vi "NewDefenderNormal.vi"(6 "Defensores":u32[](array[numeric]), 7 "total":i32, 8 "Numeric":i32, 9 "Field Size in":T3, 10 "balls":T4[](array[typedef]), 11 "Our Robot in":T1) -> (2 "Robot out":T1)   [LabVIEW 2016]
uses:
  Core/AI Robot.ctl
  Functions Enum.ctl
  Core/AI Ball.ctl
  Core/Field Size.ctl
panel:
  in  "d":dbl=110.0
  in  "min dist to kick":dbl=150.0 format="%#_13g"
  in  "D max":dbl=500.0
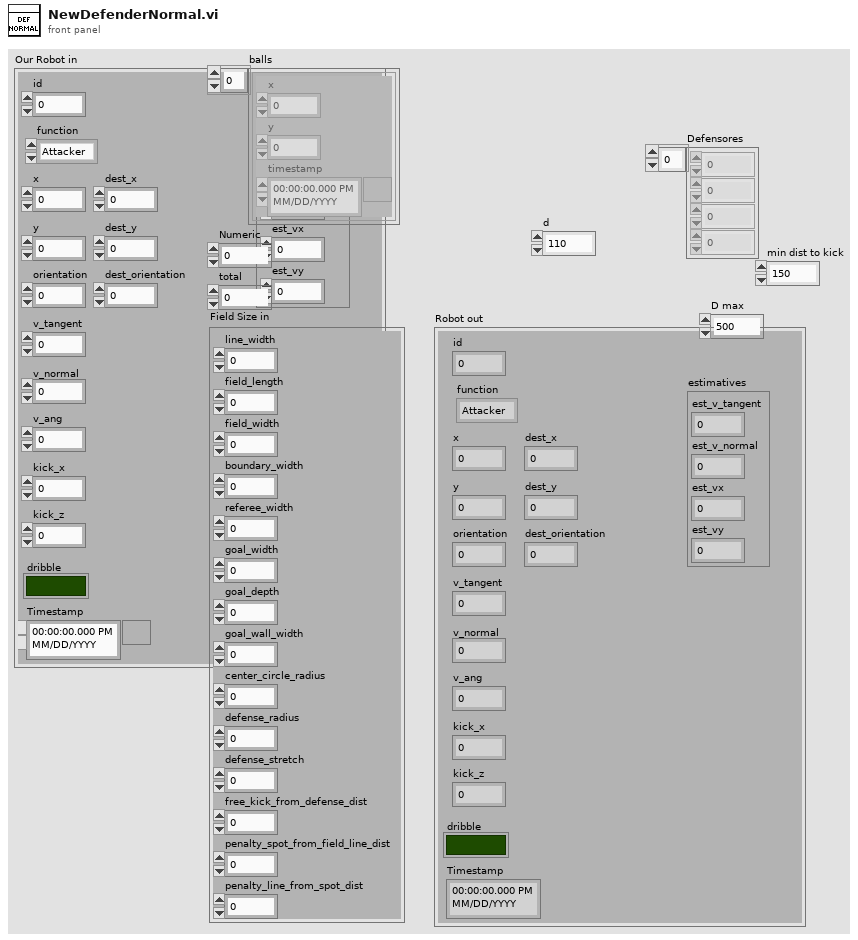
[diagram p1: front panel]
types:
  T1 = typedef "AI Robot.ctl" = cluster{"id":u32, "function":T2, "x":dbl, "y":dbl, "orientation":dbl, "v_tangent":dbl, "v_normal":dbl, "v_ang":dbl, "kick_x":dbl, "kick_z":dbl, "dribble":bool, "Timestamp":timestamp, "dest_x":dbl, "dest_y":dbl, "dest_orientation":dbl, "estimatives":cluster{"est_v_tangent":dbl, "est_v_normal":dbl, "est_vx":dbl, "est_vy":dbl}}
  T2 = typedef "Functions Enum.ctl" = enum16{"Attacker", "Goalie", "Defender", "Striker", "Goto 0", "Dummy", "ZigZag"}
  T3 = typedef "Field Size.ctl" = cluster{"line_width":u32, "field_length":u32, "field_width":u32, "boundary_width":u32, "referee_width":u32, "goal_width":u32, "goal_depth":u32, "goal_wall_width":u32, "center_circle_radius":u32, "defense_radius":u32, "defense_stretch":u32, "free_kick_from_defense_dist":u32, "penalty_spot_from_field_line_dist":u32, "penalty_line_from_spot_dist":u32}
  T4 = typedef "AI Ball.ctl" = cluster{"x":dbl, "y":dbl, "timestamp":timestamp}
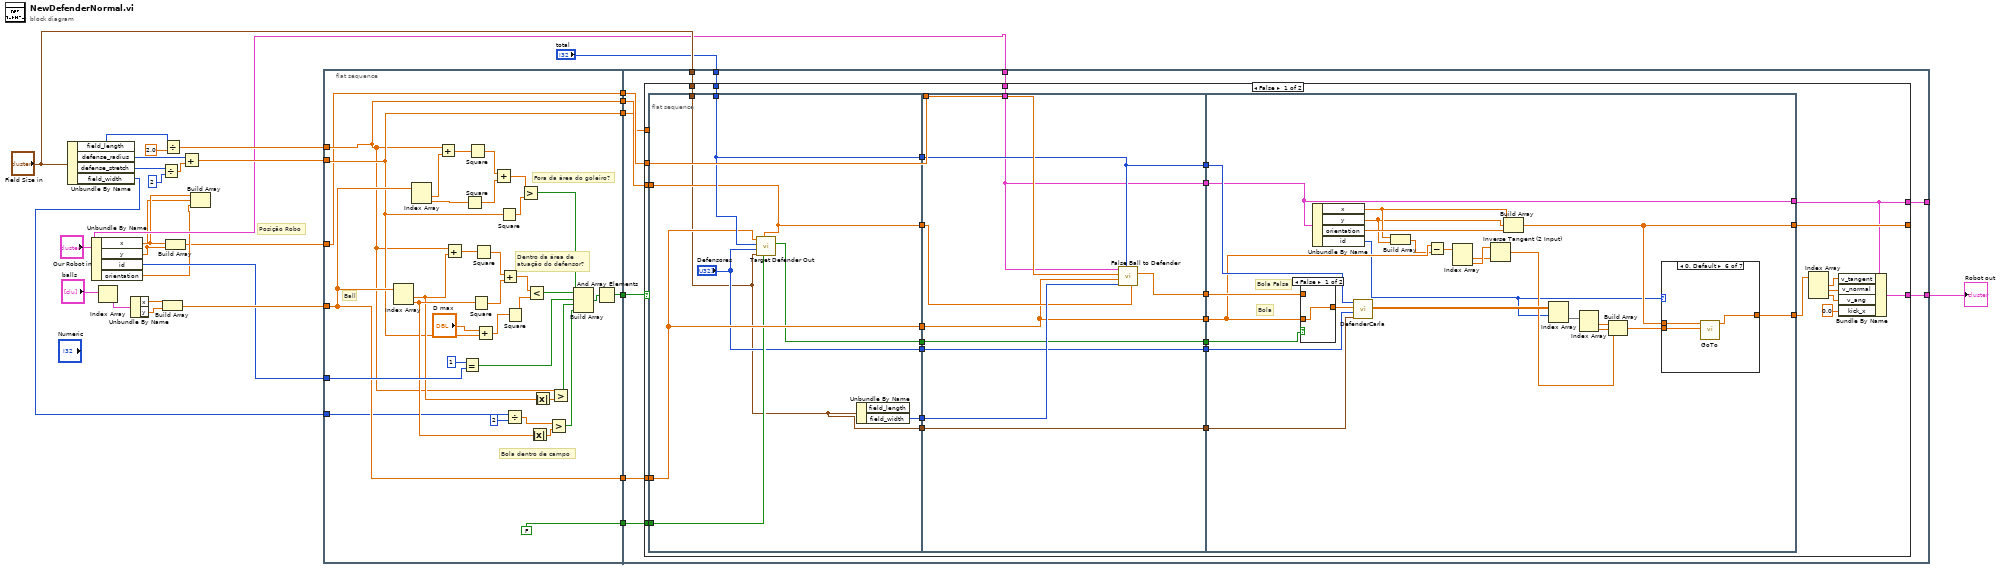
[diagram p0: block diagram]
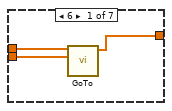
[diagram p2: hidden frame]
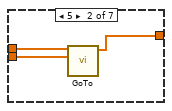
[diagram p3: hidden frame]
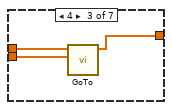
[diagram p4: hidden frame]
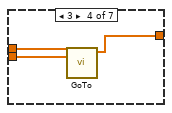
[diagram p5: hidden frame]
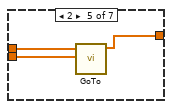
[diagram p6: hidden frame]
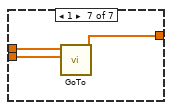
[diagram p7: hidden frame]
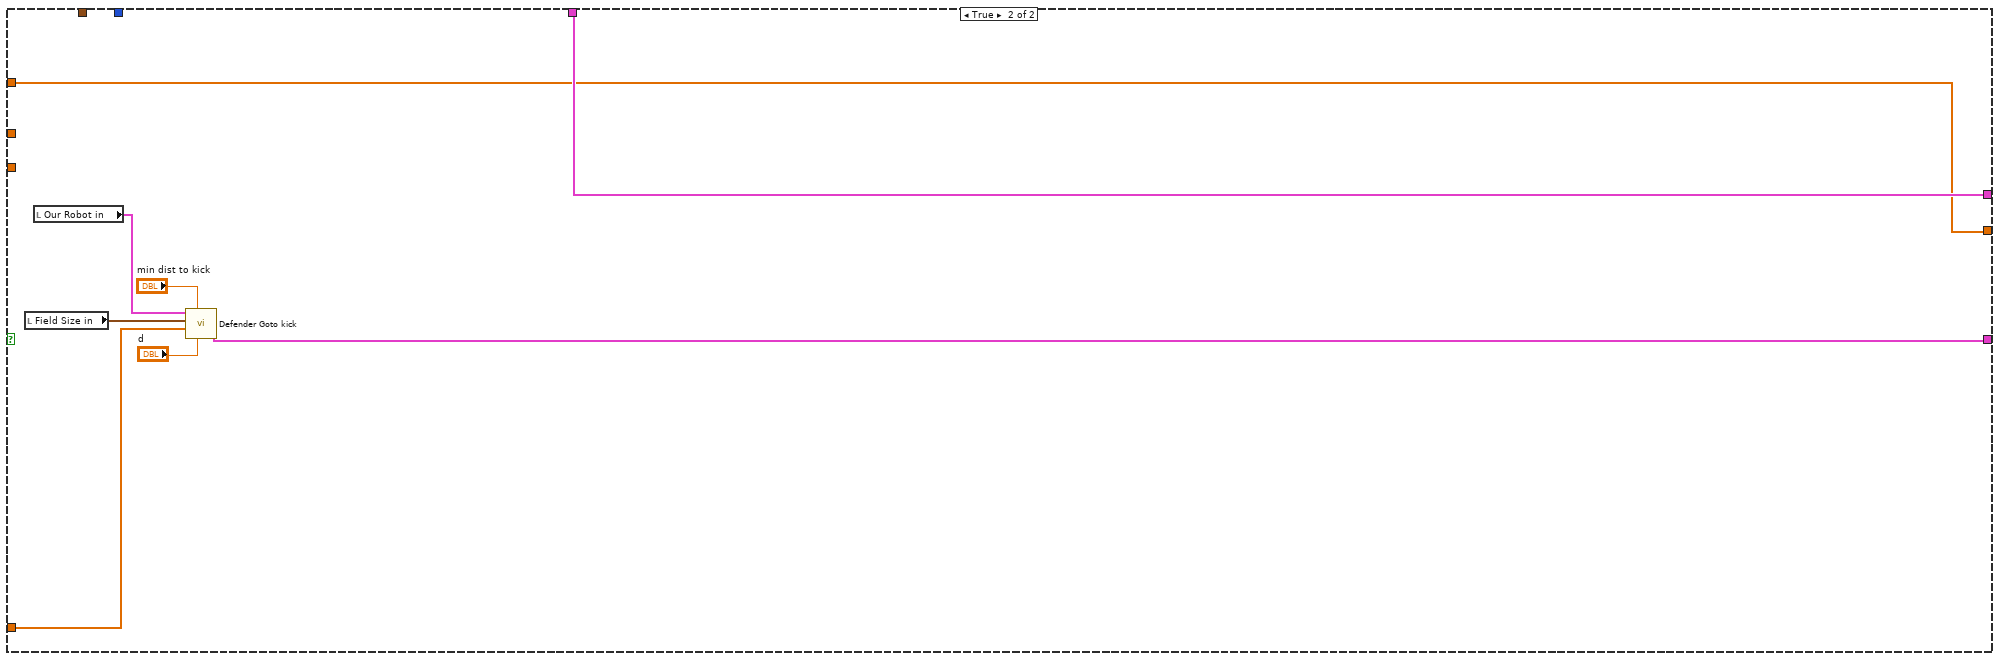
[diagram p9: hidden frame]
diagram:
  # "Posição Robo"
  n1 = Unbundle By Name("Field Size in") -> ("field_length"=w19:u32, "defense_radius"=w25:u32, "defense_stretch"=w27:u32, "field_width"=w15:u32)
  n2 = Unbundle By Name("Our Robot in") -> ("x"=w12:dbl, "y"=w11:dbl, "id"=w16:u32, "orientation"=w10:dbl)
  n3 = Index Array(array="balls") -> (element=w28:T4)  [unwired: 1 in]
  n4 = Unbundle By Name(w28) -> ("x"=w23:dbl, "y"=w22:dbl)
  n5 = Divide(x=w27, y=u32 2) -> (x/y=w26:dbl)
  n6 = Build Array(w23, w22) -> (w21:dbl[])
  n7 = Divide(x=w19, y=2.0) -> (x/y=w18:dbl)
  n8 = Build Array(w12, w11) -> (w9:dbl[])
  n9 = Add(x=w25, y=w26) -> (x+y=w17:dbl)
  n10 = Build Array(w12, w11, w10) -> ()  [unwired: 1 out]
  n11 = flat-sequence {
    tunnel: w17 -> [w32]
    tunnel: w18 -> [w31]
    tunnel: w21 -> [w48]
    tunnel: w9 -> [w30]
    tunnel: [w48] -> w8
    tunnel: [w55] -> w7
    tunnel: w16 -> [w54]
    tunnel: w15 -> [w39]
    tunnel: [FALSE ("Target Fora")] -> w6
    tunnel: [w31] -> w5
    tunnel: [w32] -> w4
    tunnel: [w30] -> w3
    tunnel: "total" -> [w75]
    tunnel: [w74] -> w1
    tunnel: w8 -> [w73]
    tunnel: w7 -> [w72]
    tunnel: w6 -> [w71]
    tunnel: w5 -> [w69]
    tunnel: "Field Size in" -> [w70]
    tunnel: "Our Robot in" -> [w68]
    tunnel: w4 -> [w67]
    tunnel: [w66] -> _
    tunnel: w3 -> [w65]
    frame #0 {
      # "Bola dentro de campo"
      # "Dentro da área de \natuação do defensor?"
      # "Fora da área do goleiro?"
      # "Ball"
      n12 = Index Array(array=w48) -> (element #1=w36:dbl, element #2=w40:dbl)  [unwired: 2 in]
      n13 = Index Array(array=w48) -> (element #1=w56:dbl, element #2=w58:dbl)  [unwired: 2 in]
      n14 = Add(x=w31, y=w56) -> (x+y=w57:dbl)
      n15 = Add(x=w31, y=w36) -> (x+y=w49:dbl)
      n16 = Equal?(x=u32 1, y=w54) -> (x = y?=w52:bool)
      n17 = Square(x=w58) -> (x^2=w60:dbl)
      n18 = Square(x=w57) -> (x^2=w59:dbl)
      n19 = Square(x=w40) -> (x^2=w51:dbl)
      n20 = Square(x=w49) -> (x^2=w50:dbl)
      n21 = Add(x="D max", y=w32) -> (x+y=w34:dbl)
      n22 = Add(x=w59, y=w60) -> (x+y=w61:dbl)
      n23 = Square(x=w32) -> (x^2=w62:dbl)
      n24 = Add(x=w50, y=w51) -> (x+y=w45:dbl)
      n25 = Divide(x=w39, y=u32 2) -> (x/y=w42:dbl)
      n26 = Square(x=w34) -> (x^2=w47:dbl)
      n27 = Greater?(x=w61, y=w62) -> (0:w63:bool)
      n28 = Less?(x=w45, y=w47) -> (x < y?=w46:bool)
      n29 = Absolute Value(x=w40) -> (abs(x)=w41:dbl)
      n30 = Absolute Value(x=w36) -> (abs(x)=w44:dbl)
      n31 = Greater?(x=w42, y=w41) -> (0:w37:bool)
      n32 = Greater?(x=w31, y=w44) -> (0:w43:bool)
      n33 = Build Array(w63, w46, w52, w43, w37) -> (w64:bool[])
      n34 = And Array Elements(Boolean array=w64) -> (logical AND=w55:bool)
    }
    frame #1 {
      n35 = case shown="False" w72 {
        tunnel: w75 -> [w103 _]
        tunnel: [w98 w177] -> w74
        tunnel: w73 -> [w97 w172]
        tunnel: w71 -> [w95 _]
        tunnel: w69 -> [w94 _]
        tunnel: w70 -> [w93 _]
        tunnel: w68 -> [w92 w171]
        tunnel: w67 -> [w91 _]
        tunnel: [w77 w170] -> _
        tunnel: [w76 w171] -> w66
        tunnel: w65 -> [_ w170]
        frame False {
          n36 = flat-sequence {
            tunnel: w103 -> [w111]
            tunnel: [w112] -> w104
            tunnel: w97 -> [w110]
            tunnel: [w111] -> w96
            tunnel: w95 -> [w108]
            tunnel: w94 -> [w109]
            tunnel: w93 -> [w105]
            tunnel: [w110] -> w90
            tunnel: [w109] -> w89
            tunnel: [w107] -> w85
            tunnel: ["Defensores"] -> w82
            tunnel: [w105] -> w80
            tunnel: w104 -> [w122]
            tunnel: w96 -> [w116]
            tunnel: w92 -> [w113]
            tunnel: w91 -> [w121]
            tunnel: w90 -> [w118]
            tunnel: w89 -> [w120]
            tunnel: [w119] -> w88
            tunnel: [w118] -> w87
            tunnel: [w117] -> w86
            tunnel: w85 -> [w117]
            tunnel: [w116] -> w84
            tunnel: [w115] -> w83
            tunnel: w82 -> [w115]
            tunnel: [w114] -> w81
            tunnel: w80 -> [w114]
            tunnel: [w113] -> w79
            tunnel: [w139] -> w78
            tunnel: [w132] -> w76
            tunnel: w88 -> [w137]
            tunnel: w87 -> [w133]
            tunnel: w86 -> [w136]
            tunnel: w84 -> [w135]
            tunnel: w83 -> [w134]
            tunnel: w81 -> [w131]
            tunnel: w79 -> [w132]
            tunnel: [w125] -> w77
            frame #0 {
              n37 = call "Target Defender Out.vi"("Target Fora in"=w108, "Campo/2"=w109, "Field Size in"=w105, "Defensores"="Defensores", "total"=w111, "Ball"=w110) -> ("Target Fora out"=w107:bool)  [unwired: 5 in]
              n38 = Unbundle By Name(w105) -> ("field_width"=w112:u32)  [unwired: 1 out]
            }
            frame #1 {
              n39 = call "False Ball to Defender.vi"("Campo/2"=w120, "field_width"=w122, "total"=w116, "Bola"=w118, "raio da área \ndo goleiro"=w121, "Our Robot in"=w113) -> ("Bola Falsa"=w119:dbl[])  [unwired: 5 in]
            }
            frame #2 {
              # "Bola"
              # "Bola Falsa"
              n40 = case shown="False" w136 {
                tunnel: [w168 w169] -> w146
                tunnel: w137 -> [_ w169]
                tunnel: w133 -> [w168 _]
                frame False {
                }
                frame True {
                }
              }
              n41 = Unbundle By Name(w132) -> ("x"=w144:dbl, "y"=w143:dbl, "orientation"=w145:dbl, "id"=w123:u32)
              n42 = call "DefenderCarla.vi"("Field Size in"=w131, "Defensores"=w134, "Ball"=w146, "total"=w135) -> ("Posição dos Defensores"=w129:dbl[][])  [unwired: 6 in]
              n43 = Build Array(w144, w143) -> (w130:dbl[])
              n44 = Subtract(x=w133, y=w130) -> (x-y=w142:dbl[])
              n45 = Index Array(array=w142) -> (element #1=w140:dbl, element #2=w141:dbl)  [unwired: 2 in]
              n46 = Inverse Tangent (2 Input)(1:w140, 2:w141) -> (0:w124:dbl)
              n47 = Build Array(w144, w143, w145) -> (w125:dbl[])
              n48 = Index Array(array=w129, index (row)=w123) -> (element=w128:dbl[])  [unwired: 1 in]
              n49 = Index Array(array=w128) -> (element #1=w127:dbl, element #2=w126:dbl)  [unwired: 2 in]
              n50 = Build Array(w127, w126, w124) -> (w138:dbl[])
              n51 = case shown="0, Default" w123 {
                tunnel: [w147 w150 w153 w156 w159 w162 w167] -> w139
                tunnel: w138 -> [w148 w152 w154 w157 w160 w163 w166]
                tunnel: w125 -> [w149 w151 w155 w158 w161 w164 w165]
                frame 6 {
                  n52 = call "GoTo.vi"("Target"=w148, "Position"=w149) -> ("Output\nVelocity"=w147:dbl[])  [unwired: 8 in, 1 out]
                }
                frame 5 {
                  n53 = call "GoTo.vi"("Target"=w152, "Position"=w151) -> ("Output\nVelocity"=w150:dbl[])  [unwired: 8 in, 1 out]
                }
                frame 4 {
                  n54 = call "GoTo.vi"("Target"=w154, "Position"=w155) -> ("Output\nVelocity"=w153:dbl[])  [unwired: 8 in, 1 out]
                }
                frame 3 {
                  n55 = call "GoTo.vi"("Target"=w157, "Position"=w158) -> ("Output\nVelocity"=w156:dbl[])  [unwired: 8 in, 1 out]
                }
                frame 2 {
                  n56 = call "GoTo.vi"("Target"=w160, "Position"=w161) -> ("Output\nVelocity"=w159:dbl[])  [unwired: 8 in, 1 out]
                }
                frame 0, Default {
                  n57 = call "GoTo.vi"("Target"=w163, "Position"=w164) -> ("Output\nVelocity"=w162:dbl[])  [unwired: 8 in, 1 out]
                }
                frame 1 {
                  n58 = call "GoTo.vi"("Target"=w166, "Position"=w165) -> ("Output\nVelocity"=w167:dbl[])  [unwired: 8 in, 1 out]
                }
              }
            }
          }
          n59 = Index Array(array=w78) -> (element #1=w101:dbl, element #2=w100:dbl, element #3=w99:dbl)  [unwired: 3 in]
          n60 = Bundle By Name(cluster=w76, "v_tangent"=w101, "v_normal"=w100, "v_ang"=w99, "kick_x"=0.0) -> (w98:T1)
        }
        frame True {
          n61 = local read "Field Size in"() -> (w175:T3)
          n62 = local read "Our Robot in"() -> (w176:T1)
          n63 = call "Defender Goto kick.vi"("d"="d", "min dist to kick"="min dist to kick", "Bola"=w172, "Field Size in"=w175, "Our Robot in"=w176) -> ("Our Robot out"=w177:T1)  [unwired: 6 in]
        }
      }
    }
  }
  "Robot out" <- w1
